vi "GA Set Soft Limit.vi"(8 "error in (no error)":errorcluster caption="错误输入（无错误）", 9 "lNegative":i32, 10 "lPositive":i32, 11 "nAxisNum":i16) -> (0 "error out":errorcluster caption="错误输出", 3 "function return":i32)   [LabVIEW 2024, in "GAS.lvlib"]
doc: "extern \"C\" __declspec(dllimport) int GA_SetSoftLimit(short nAxisNum,long lPositive,long lNegative);"
uses:
  GAS.lvlib
  GAS.dll
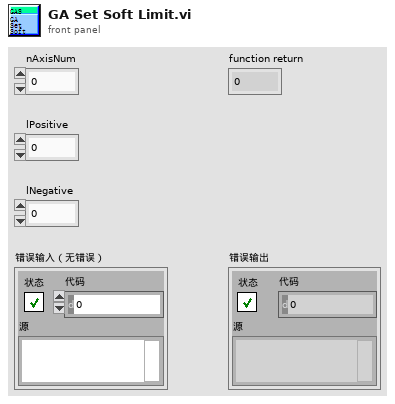
[diagram p1: front panel]
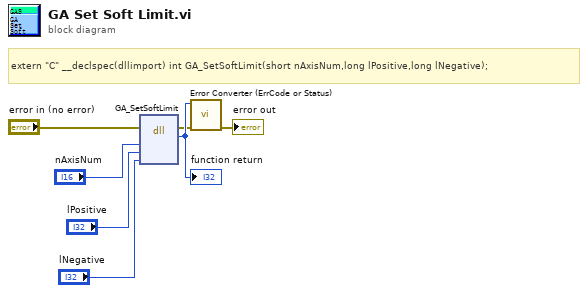
[diagram p0: block diagram]
diagram:
  # "extern \"C\" __declspec(dllimport) int GA_SetSoftLimit(short nAxisNum,long lPositive,long lNegative);"
  n1 = dll-call lib="PTH2?abs D实验室软件（勿删）集成测试系统GAS.*" fn="GA_SetSoftLimit"(error in="error in (no error)", "nAxisNum"="nAxisNum", "lPositive"="lPositive", "lNegative"="lNegative") -> (error out=w2:errorcluster, w7:i32)  [unwired: 5 in, 1 out]
  "function return" <- w7
  n2 = call "Error Converter (ErrCode or Status).vi"("error in (no error)"=w2, "error code"=w7) -> ("error out"=→"error out":errorcluster)  [unwired: 9 in]
